vi "SUB_Del_SpecificFile_inAnyFolder.vi"(4 "filename to be deleted":string="Fl7.cfg", 5 "Base path":string) -> (2 "error code":i32)   [LabVIEW 2011]
panel:
  out "concatenated string":string
  out "error out 2":errorcluster
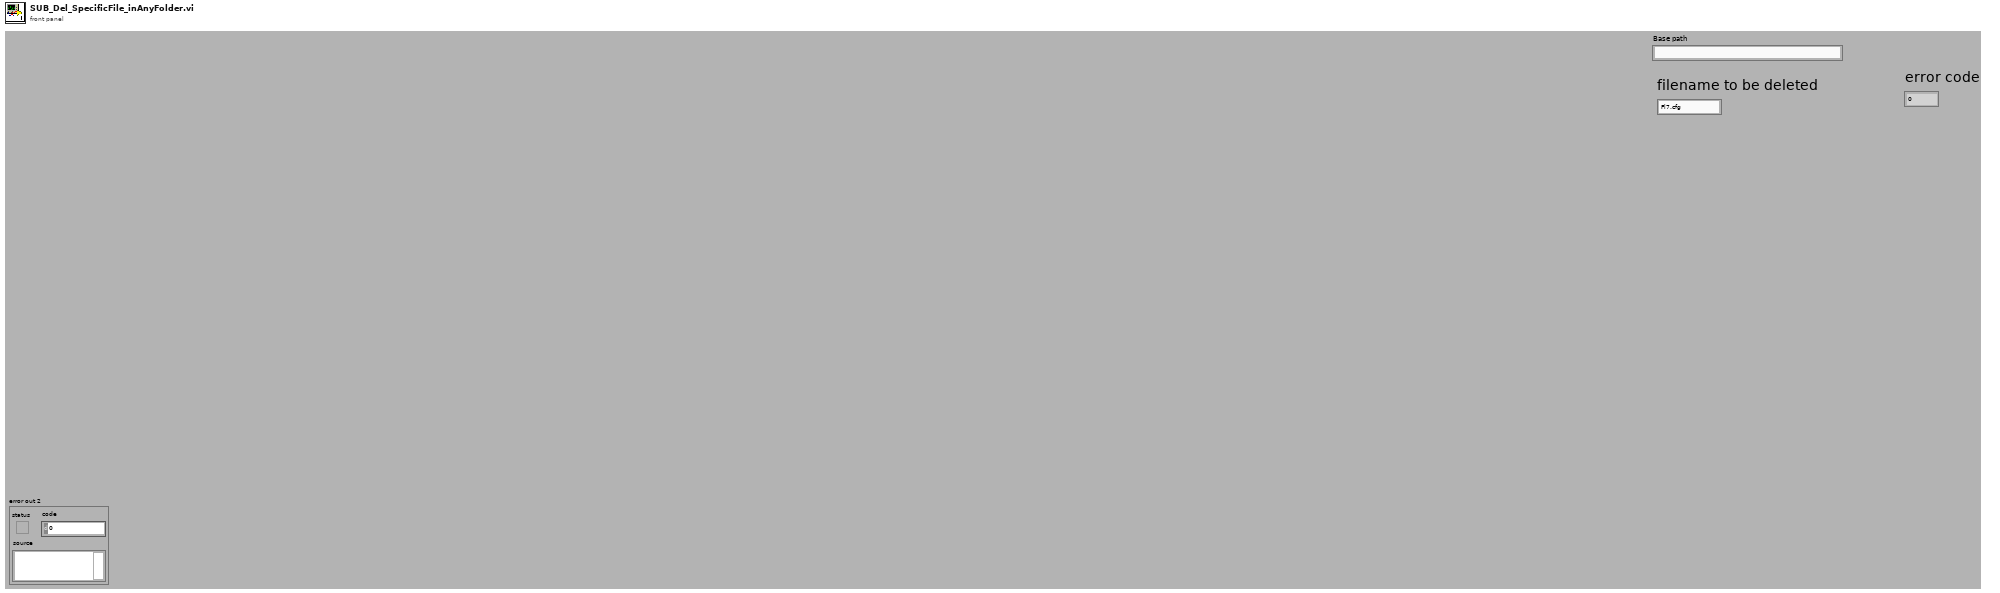
[diagram p1: front panel]
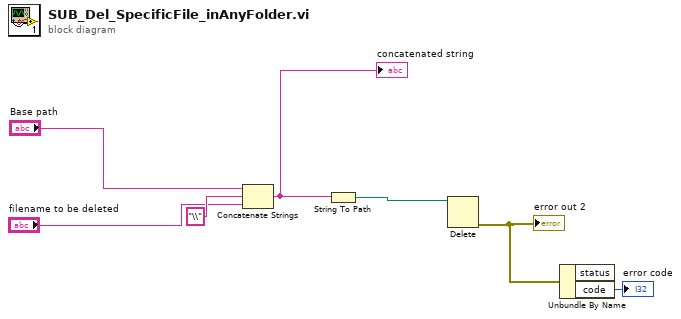
[diagram p0: block diagram]
diagram:
  n1 = Concatenate Strings("Base path", "\\" ("string"), "filename to be deleted") -> (w6:string)
  "concatenated string" <- w6
  n2 = String To Path(string=w6) -> (path=w5:path)
  n3 = Delete(path (use dialog)=w5) -> (error out=w3:errorcluster)  [unwired: 4 in, 2 out]
  "error out 2" <- w3
  n4 = Unbundle By Name(w3) -> ("code"=→"error code":i32)  [unwired: 1 out]
